vi "process.vi"(8 "error in (no error)":errorcluster, 11 "Default in":refnum<class "Default.lvclass">) -> (0 "error out":errorcluster, 3 "Default out":refnum<class "Default.lvclass">)   [LabVIEW 2016, in "Default.lvclass"]
uses:
  Default.lvclass
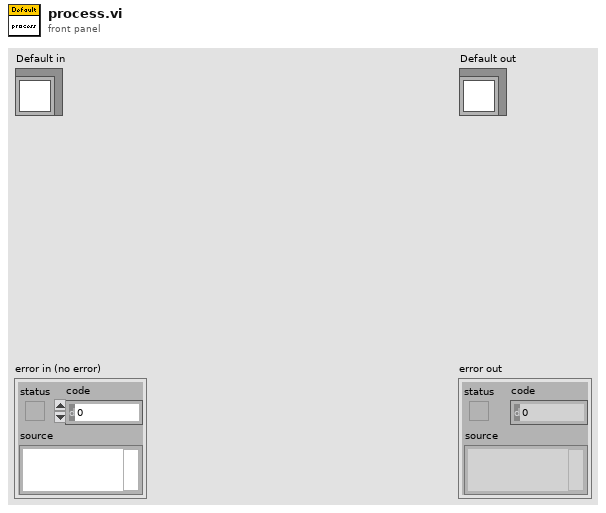
[diagram p1: front panel]
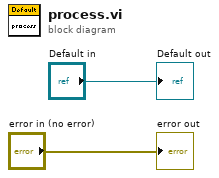
[diagram p0: block diagram]
diagram:
  "error out" <- "error in (no error)"
  "Default out" <- "Default in"
